vi "ControlCam-Final.vi"() -> ()   [LabVIEW 2014]
uses:
  <vilib>/vision/Vision Builder AI/API.llb/IVB Interface - VBAI Version.ctl
  <vilib>/vision/Vision Builder AI/API.llb/VBAI Interface - Get Inspection Image (By Name).vi
panel:
  out "Illegal?":bool
  out "Goal?":bool
  out "XY Graph":cluster{dbl[], dbl[]}[](graph)
  out "Ymovement":dbl
  out "X movefromcenter":dbl
  out "THETA case(deg)":dbl
  out "Defence 2 X":dbl format="%_4g"
  out "Defence 2 Y":dbl format="%_4g"
  in  "Kick":bool
  out "Defender 2":bool
  in  "Reset":bool
  out "Defender 1":bool
  out "Defenders":dbl
  out "MatchBall?":bool
  out "No.OfMatchball":dbl
  out "No.OfKicker":dbl
  out "Kicker There ?":bool
  out "Defence 1 Y":dbl format="%_4g"
  out "Defence 1 X":dbl format="%_4g"
  out "MatchBall Y":dbl format="%_4g"
  out "MatchBallX":dbl format="%_4g"
  out "Kicker Y":dbl format="%_4g"
  out "Kicker X":dbl format="%_4g"
  out "Image":T1(plugin-control)
  in  "stop":bool
  # "Manish's Free Kick Kicker"
  # "Co-ordinates in Centimeters"
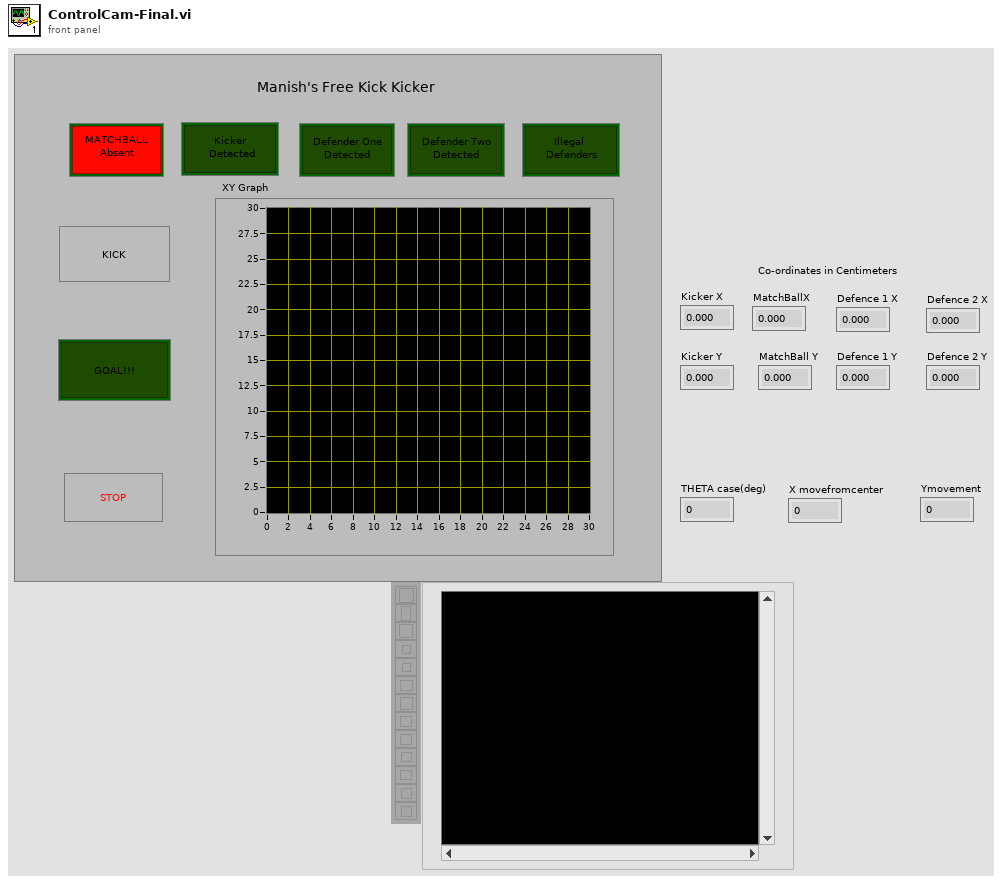
[diagram p1: front panel]
types:
  T1 = typedef "IMAQ Image.ctl" = refnum<image>
  T2 = typedef "Image Type" = u32
  T3 = typedef "IVB Interface - VBAI Version.ctl" = u16
  T4 = typedef "VBAIInterface.ctl" = refnum<k21>
  T5 = cluster{"PASS/FAIL Flag":bool, "Numeric Measurement":dbl, "String Measurement":string, "Report Text":string}[]
  T6 = cluster{"PASS/FAIL Flag":bool, "Numeric Measurement":dbl, "String Measurement":string, "Report Text":string}
  T7 = cluster{"m":dbl, "MatchBallX":dbl, "type":dbl, "MatchBallY":dbl}
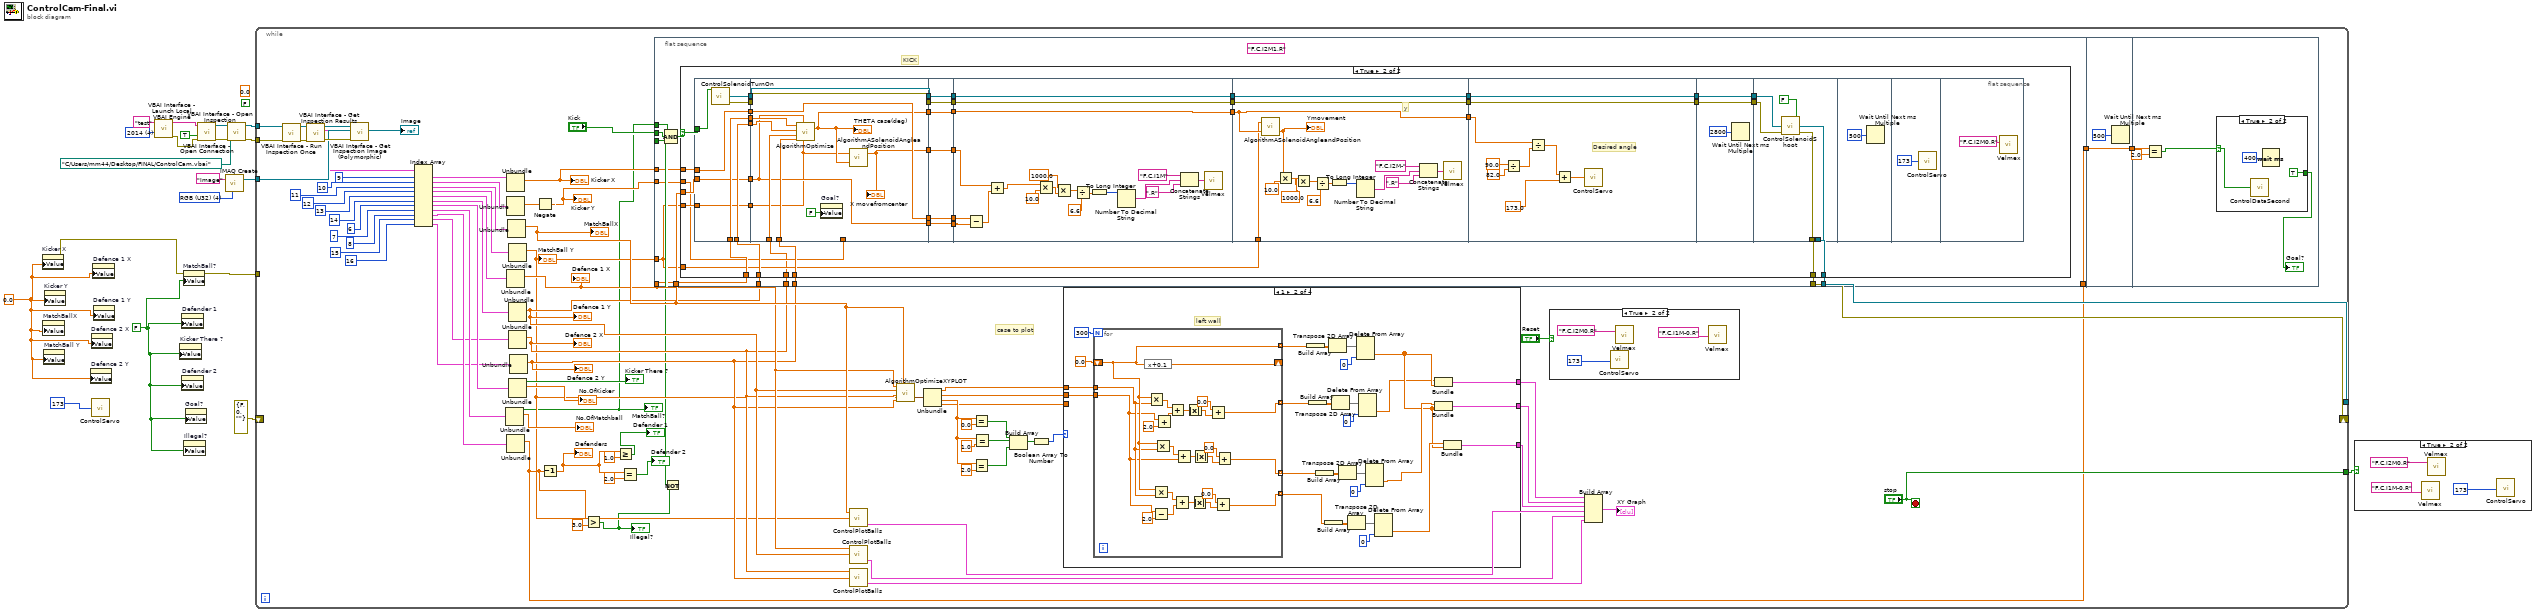
[diagram p0: block diagram]
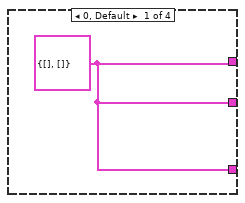
[diagram p3: hidden frame]
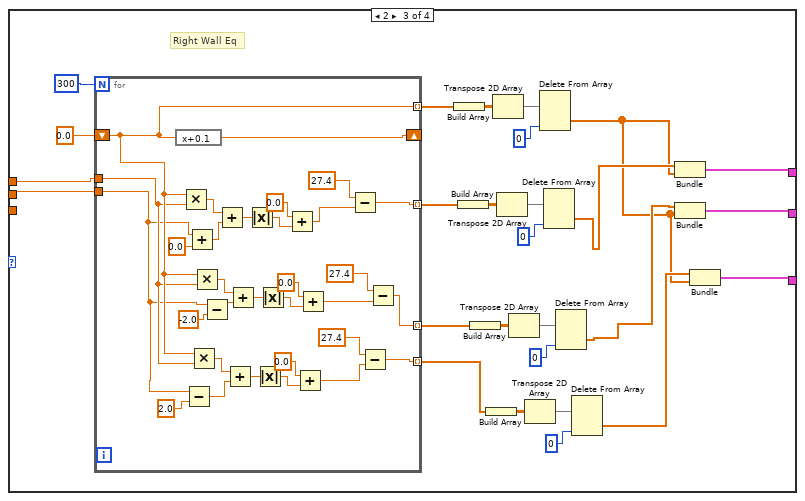
[diagram p4: hidden frame]
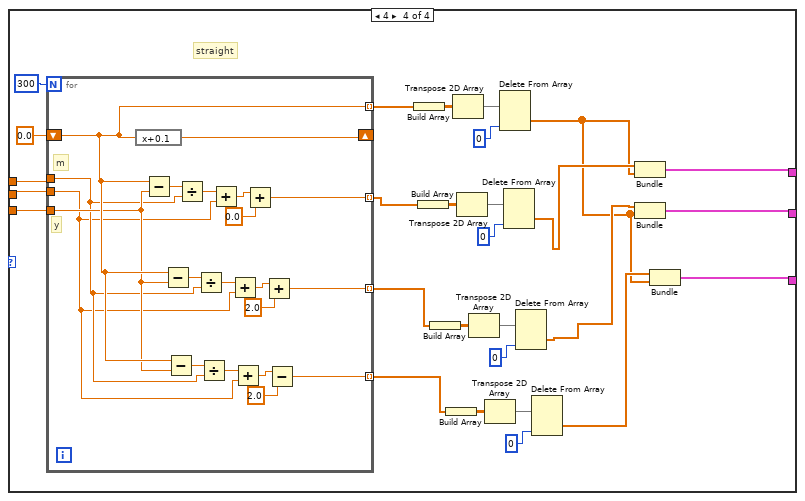
[diagram p5: hidden frame]
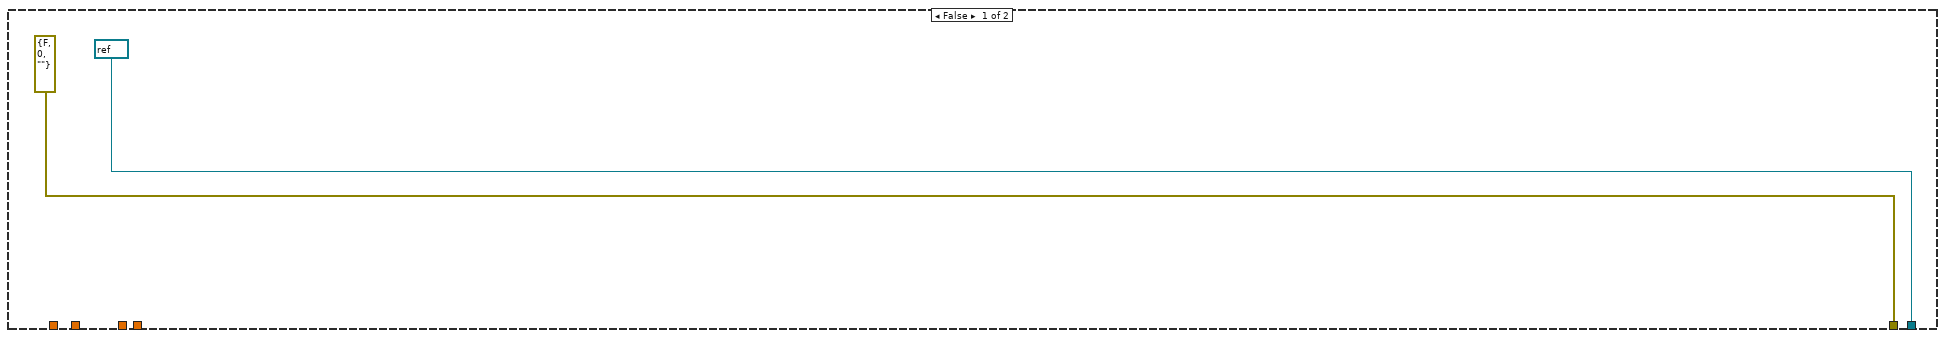
[diagram p6: hidden frame]
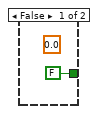
[diagram p7: hidden frame]
diagram:
  (unwired) FALSE
  (unwired) 0.0
  w3 = 0.0 ("Kicker X")
  w1 = FALSE
  w9 = T2 4 items=["Grayscale (U8)", "Grayscale (I16)", "Grayscale (SGL)", "Complex (CSG)", "RGB (U32)", "HSL (U32)", "RGB (U64)", "Grayscale (U16)"] ("Image Type")
  w17 = T3 4 items=["2010", "2011", "2012", "2013", "2014"] ("Engine Version")
  n1 = property on="Kicker X" class="DigNum (strict)"("Value"=w3) -> (error out=w4:errorcluster)  [unwired: 2 in, 1 out]
  n2 = property on="MatchBallX" class="DigNum (strict)"("Value"=w3) -> ()  [unwired: 2 in, 2 out]
  n3 = property on="MatchBall Y" class="DigNum (strict)"("Value"=w3) -> ()  [unwired: 2 in, 2 out]
  n4 = property on="Kicker Y" class="DigNum (strict)"("Value"=w3) -> ()  [unwired: 2 in, 2 out]
  n5 = property on="Defence 2 Y" class="DigNum (strict)"("Value"=w3) -> ()  [unwired: 2 in, 2 out]
  n6 = property on="Defence 2 X" class="DigNum (strict)"("Value"=w3) -> ()  [unwired: 2 in, 2 out]
  n7 = call "ControlServo.vi"("position"=u8 173) -> ()
  n8 = property on="Defence 1 X" class="DigNum (strict)"("Value"=w3) -> ()  [unwired: 2 in, 2 out]
  n9 = property on="Defence 1 Y" class="DigNum (strict)"("Value"=w3) -> ()  [unwired: 2 in, 2 out]
  n10 = call <vilib>:"VBAI Interface - Launch Local VBAI Engine.vi"("Engine Version"=w17, "Local VBAI Engine Name"="test") -> ("error out"=w8:errorcluster, "Session Name Out"=w18:string)  [unwired: 8 in]
  n11 = property on="Kicker There ?" class="Bool (strict)"("Value"=w1) -> ()  [unwired: 2 in, 2 out]
  n12 = property on="Defender 1" class="Bool (strict)"("Value"=w1) -> ()  [unwired: 2 in, 2 out]
  n13 = property on="Defender 2" class="Bool (strict)"("Value"=w1) -> ()  [unwired: 2 in, 2 out]
  n14 = property on="MatchBall?" class="Bool (strict)"(error in=w4, "Value"=w1) -> (error out=w7:errorcluster)  [unwired: 1 in, 1 out]
  n15 = property on="Illegal?" class="Bool (strict)"("Value"=w1) -> ()  [unwired: 2 in, 2 out]
  n16 = property on="Goal?" class="Bool (strict)"("Value"=w1) -> ()  [unwired: 2 in, 2 out]
  n17 = call <vilib>:"VBAI Interface - Open Connection.vi"("error in"=w8, "Force Connection (False)"=TRUE, "Session In"=w18) -> ("error out"=w16:errorcluster, "Session Out"=w15:T4)  [unwired: 7 in]
  n18 = call "IMAQ Create"("Image Name"="Image", "Image Type"=w9) -> ("New Image"=w11:T1)  [unwired: 3 in, 1 out]
  n19 = call <vilib>:"VBAI Interface - Open Inspection.vi"("error in"=w16, "Path"=path "C:/Users/mm44/Desktop/FINAL/ControlCam.vbai", "Session In"=w15) -> ("error out"=w12:errorcluster, "Session Out"=w13:T4)  [unwired: 7 in]
  n20 = while {
    tunnel: w13 -> [w98]
    tunnel: w12 -> [w97]
    tunnel: w11 -> [w94]
    tunnel: w7 -> [_]
    shift-right: [w57] -> _
    shift-left: errorcluster {"status"=FALSE, "code"=0, "source"=""} ("error out") -> [_]
    tunnel: [w58] -> _
    tunnel: ["stop"] -> w5
    stop <- "stop" stop-if-true
    # "case to plot"
    n21 = call <vilib>:"VBAI Interface - Run Inspection Once.vi"("error in"=w97, "Session In"=w98) -> ("error out"=w100:errorcluster, "Session Out"=w99:T4)  [unwired: 8 in]
    n22 = call <vilib>:"VBAI Interface - Get Inspection Results.vi"("error in"=w100, "Session In"=w99) -> ("error out"=w95:errorcluster, "Step Results"=w92:T5, "Session Out"=w96:T4)  [unwired: 3 in, 4 out]
    n23 = call-poly <vilib>:"VBAI Interface - Get Inspection Image (Polymorphic).vi"("error in"=w95, "Image Dest"=w94, "Session In"=w96) -> ("Image Dst Out"=→"Image":T1)  [unwired: 5 in, 3 out]
    n24 = Index Array(array=w92, index #1=9 ("index"), index #2=10 ("index"), index #3=11 ("index"), index #4=12 ("index"), index #5=13 ("index"), index #6=14 ("index"), index #7=6 ("index"), index #8=7 ("index"), index #9=8 ("index"), index #10=15 ("index"), index #11=16 ("index")) -> (element #1=w91:T6, element #2=w89:T6, element #3=w82:T6, element #4=w81:T6, element #5=w80:T6, element #6=w79:T6, element #7=w77:T6, element #8=w73:T6, element #9=w71:T6, element #10=w62:T6, element #11=w61:T6)
    n25 = Unbundle(w73) -> ("PASS/FAIL Flag"=w25:bool, "Numeric Measurement"=→"No.OfMatchball":dbl)  [unwired: 2 out]
    "MatchBall?" <- w25
    n26 = Unbundle(w91) -> ("Numeric Measurement"=w52:dbl)  [unwired: 3 out]
    "Kicker X" <- w52
    n27 = Unbundle(w89) -> ("Numeric Measurement"=w88:dbl)  [unwired: 3 out]
    n28 = Unbundle(w80) -> ("Numeric Measurement"=w36:dbl)  [unwired: 3 out]
    "Defence 1 X" <- w36
    n29 = Unbundle(w71) -> ("Numeric Measurement"=w23:dbl)  [unwired: 3 out]
    n30 = Unbundle(w82) -> ("Numeric Measurement"=w37:dbl)  [unwired: 3 out]
    "MatchBallX" <- w37
    n31 = Unbundle(w81) -> ("Numeric Measurement"=w32:dbl)  [unwired: 3 out]
    "MatchBall Y" <- w32
    n32 = Unbundle(w79) -> ("Numeric Measurement"=w35:dbl)  [unwired: 3 out]
    "Defence 1 Y" <- w35
    n33 = Unbundle(w62) -> ("Numeric Measurement"=w34:dbl)  [unwired: 3 out]
    "Defence 2 X" <- w34
    n34 = Unbundle(w77) -> ("PASS/FAIL Flag"=→"Kicker There ?":bool, "Numeric Measurement"=→"No.OfKicker":dbl)  [unwired: 2 out]
    n35 = Unbundle(w61) -> ("Numeric Measurement"=w33:dbl)  [unwired: 3 out]
    "Defence 2 Y" <- w33
    n36 = Negate(x=w88) -> (-x=w51:dbl)
    "Kicker Y" <- w51
    n37 = Decrement(x=w23) -> (x-1=w65:dbl)
    "Defenders" <- w65
    n38 = Greater?(x=w23, y=3.0) -> (0:w22:bool)
    "Illegal?" <- w22
    n39 = Greater Or Equal?(x=w65, y=1.0) -> (x >= y?=→"Defender 1":bool)
    n40 = Equal?(x=w65, y=2.0) -> (x = y?=→"Defender 2":bool)
    n41 = flat-sequence {
      tunnel: "Kick" -> [w260]
      tunnel: [w272] -> w58
      tunnel: [w271] -> w57
      tunnel: w52 -> [w270]
      tunnel: w51 -> [w269]
      tunnel: w37 -> [w268]
      tunnel: w32 -> [w267]
      tunnel: w36 -> [w266]
      tunnel: w35 -> [w265]
      tunnel: w34 -> [w264]
      tunnel: w33 -> [w263]
      tunnel: w23 -> [w262]
      tunnel: [w262] -> w26
      tunnel: w25 -> [w261]
      tunnel: w21 -> [w258]
      tunnel: [w397] -> w27
      tunnel: w26 -> [w397]
      tunnel: w27 -> [w402]
      frame #0 {
        (unwired) "F,C,I2M1,R" ("string")
        # "KICK"
        n42 = Compound Arithmetic op=AND(w261, w260, w258) -> (w259:bool)
        n43 = case shown="True" w259 {
          selector: w259 -> [_ w311]
          tunnel: w268 -> [_ w315]
          tunnel: w267 -> [_ w281]
          tunnel: w270 -> [_ w314]
          tunnel: [refnum<k21> refnum ("task out") w313] -> w272
          tunnel: [errorcluster {"status"=FALSE, "code"=0, "source"=""} ("error out") w312] -> w271
          tunnel: w266 -> [_ w301]
          tunnel: w265 -> [_ w300]
          tunnel: w264 -> [_ w275]
          tunnel: w263 -> [_ w298]
          tunnel: w269 -> [_ w277]
          tunnel: w267 -> [_ w276]
          frame False {
          }
          frame True {
            n44 = flat-sequence {
              tunnel: w314 -> [w317]
              tunnel: w315 -> [w318]
              tunnel: [w318] -> w306
              tunnel: [w317] -> w305
              tunnel: w311 -> [w323]
              tunnel: [w322] -> w304
              tunnel: [w321] -> w303
              tunnel: [w320] -> w302
              tunnel: w301 -> [w320]
              tunnel: w300 -> [w319]
              tunnel: [w319] -> w299
              tunnel: [w316] -> w282
              tunnel: w281 -> [w316]
              tunnel: w306 -> [w328]
              tunnel: [w328] -> w297
              tunnel: w305 -> [w333]
              tunnel: [w333] -> w296
              tunnel: w304 -> [w335]
              tunnel: [w335] -> w294
              tunnel: w303 -> [w334]
              tunnel: [w334] -> w292
              tunnel: w302 -> [w332]
              tunnel: w299 -> [w331]
              tunnel: w275 -> [w330]
              tunnel: w298 -> [w329]
              tunnel: [w327] -> w290
              tunnel: w282 -> [w324]
              tunnel: [w326] -> w280
              tunnel: w277 -> [_]
              tunnel: w297 -> [w337]
              tunnel: w296 -> [w341]
              tunnel: [w341] -> w295
              tunnel: w294 -> [w340]
              tunnel: [w340] -> w293
              tunnel: w292 -> [w339]
              tunnel: [w339] -> w291
              tunnel: w290 -> [w338]
              tunnel: [w338] -> w289
              tunnel: [w337] -> w283
              tunnel: w280 -> [w336]
              tunnel: [w336] -> w279
              tunnel: w295 -> [w347]
              tunnel: [w350] -> w288
              tunnel: w293 -> [w350]
              tunnel: [w349] -> w286
              tunnel: w291 -> [w349]
              tunnel: [w348] -> w284
              tunnel: w289 -> [w348]
              tunnel: w283 -> [w346]
              tunnel: w279 -> [w343]
              tunnel: w288 -> [w376]
              tunnel: [w376] -> w287
              tunnel: w286 -> [w375]
              tunnel: [w375] -> w285
              tunnel: w284 -> [w362]
              tunnel: [w362] -> w278
              tunnel: w276 -> [w361]
              tunnel: [w385] -> w309
              tunnel: w287 -> [w385]
              tunnel: [w384] -> w307
              tunnel: w285 -> [w384]
              tunnel: w278 -> [w381]
              tunnel: [w388] -> w310
              tunnel: w309 -> [w388]
              tunnel: [w387] -> w308
              tunnel: w307 -> [w387]
              tunnel: [w392] -> w313
              tunnel: [w391] -> w312
              tunnel: w310 -> [w390]
              tunnel: w308 -> [w389]
              frame #0 {
                n45 = call "ControlSolenoidTurnOn.vi"("On?"=w323) -> ("error out"=w321:errorcluster, "task out"=w322:refnum<k21>)
              }
              frame #1 {
                n46 = call "AlgorithmOptimize.vi"("MatchBallY"=w324, "MatchBallX"=w328, "D2 Y COM"=w329, "D2 X COM"=w330, "D1Y COM"=w331, "D1 X COM 2"=w332) -> ("THETA"=w327:dbl)  [unwired: 1 in]
                "THETA case(deg)" <- w327
                n47 = property on="Goal?" class="Bool (strict)"("Value"=FALSE ("Goal?")) -> ()  [unwired: 2 in, 2 out]
                n48 = call "AlgorithmASolenoidAngleandPosition.vi"("Theta in degrees"=w327, "MartchBall Y"=w324) -> ("X movefromcenter"=w326:dbl)  [unwired: 1 out]
                "X movefromcenter" <- w326
              }
              frame #2 {
              }
              frame #3 {
                n49 = Subtract(x=w347, y=w346) -> (x-y=w344:dbl)
                n50 = Add(x=w343, y=w344) -> (x+y=w345:dbl)
                n51 = Multiply(x=w345, y=10.0) -> (x*y=w357:dbl)
                n52 = Multiply(x=1000.0, y=w357) -> (x*y=w355:dbl)
                n53 = Divide(x=w355, y=6.6) -> (x/y=w342:dbl)
                n54 = To Long Integer(number=w342) -> (32bit integer=w353:i32)
                n55 = Number To Decimal String(number=w353) -> (decimal integer string=w352:string)  [unwired: 1 in]
                n56 = Concatenate Strings("F,C,I1M" ("string"), w352, ",R" ("string")) -> (w351:string)
                n57 = call "Velmex.Vi"("Command String"=w351) -> ()  [unwired: 6 in]
              }
              frame #4 {
                # "y"
                n58 = call "AlgorithmASolenoidAngleandPosition.vi"("Theta in degrees"=w362, "MartchBall Y"=w361) -> ("Ymovement"=w363:dbl)  [unwired: 1 out]
                "Ymovement" <- w363
                n59 = Multiply(x=w363, y=10.0) -> (x*y=w367:dbl)
                n60 = Multiply(x=1000.0, y=w367) -> (x*y=w369:dbl)
                n61 = Divide(x=w369, y=6.6) -> (x/y=w371:dbl)
                n62 = To Long Integer(number=w371) -> (32bit integer=w372:i32)
                n63 = Number To Decimal String(number=w372) -> (decimal integer string=w373:string)  [unwired: 1 in]
                n64 = Concatenate Strings("F,C,I2M-" ("string"), w373, ",R" ("string")) -> (w374:string)
                n65 = call "Velmex.Vi"("Command String"=w374) -> ()  [unwired: 6 in]
              }
              frame #5 {
                # "Desired angle"
                n66 = Divide(x=90.0, y=82.0) -> (x/y=w380:dbl)
                n67 = Divide(x=w381, y=w380) -> (x/y=w379:dbl)
                n68 = Add(x=w379, y=173.0) -> (x+y=w377:dbl)
                n69 = call "ControlServo.vi"("position"=w377) -> ()
              }
              frame #6 {
                n70 = Wait Until Next ms Multiple(millisecond multiple=u32 2800) -> ()  [unwired: 1 out]
              }
              frame #7 {
                n71 = call "ControlSolenoidShoot.vi"("error in"=w389, "task/channels in"=w390, "On?"=FALSE) -> ("error out"=w391:errorcluster, "task out"=w392:refnum<k21>)  [unwired: 1 in]
              }
              frame #8 {
                n72 = Wait Until Next ms Multiple(millisecond multiple=u32 500) -> ()  [unwired: 1 out]
              }
              frame #9 {
                n73 = call "ControlServo.vi"("position"=173) -> ()
              }
              frame #10 {
                n74 = call "Velmex.Vi"("Command String"="F,C,I2M0,R" ("Y 2")) -> ()  [unwired: 6 in]
              }
            }
          }
        }
      }
      frame #1 {
        n75 = Wait Until Next ms Multiple(millisecond multiple=u32 500) -> ()  [unwired: 1 out]
      }
      frame #2 {
        n76 = Equal?(x=w402, y=2.0) -> (x = y?=w400:bool)
        n77 = case shown="True" w400 {
          selector: w400 -> [_ w404]
          tunnel: [FALSE TRUE] -> w399
          frame False {
            (unwired) 0.0
          }
          frame True {
            n78 = call "ControlDataSecond.vi"("Boolean"=w404) -> ()  [unwired: 2 in]
            n79 = Wait (ms)(milliseconds to wait=u32 400) -> ()  [unwired: 1 out]
          }
        }
        "Goal?" <- w399
      }
    }
    n80 = Not(x=w22) -> (.not. x?=w21:bool)
    n81 = call "ControlPlotBalls.vi"("Y-center"=w32, "x-center"=w37) -> ("XY Graph"=w55:cluster{dbl[], dbl[]})
    n82 = call "ControlPlotBalls.vi"("Y-center"=w35, "x-center"=w36) -> ("XY Graph"=w54:cluster{dbl[], dbl[]})
    n83 = call "ControlPlotBalls.vi"("Y-center"=w33, "x-center"=w34) -> ("XY Graph"=w50:cluster{dbl[], dbl[]})
    n84 = call "AlgorithmOptimizeXYPLOT.vi"("MatchBallY"=w32, "MatchBallX"=w37, "D2 Y COM"=w33, "D2 X COM"=w34, "D1Y COM"=w35, "D1 X COM 2"=w36) -> ("Plot"=w49:T7)  [unwired: 1 out]
    n85 = Unbundle(w49) -> ("m"=w40:dbl, "MatchBallX"=w39:dbl, "type"=w45:dbl, "MatchBallY"=w38:dbl)
    n86 = Equal?(x=w45, y=0.0) -> (x = y?=w46:bool)
    n87 = Equal?(x=w45, y=2.0) -> (x = y?=w42:bool)
    n88 = Equal?(x=w45, y=1.0) -> (x = y?=w43:bool)
    n89 = Build Array(w46, w43, w42) -> (w47:bool[])
    n90 = Boolean Array To Number(Boolean array=w47) -> (number=w41:u32)
    n91 = case shown="1" w41 {
      tunnel: w40 -> [_ w107 w156 w217]
      tunnel: w39 -> [_ w106 w155 w216]
      tunnel: w38 -> [_ _ _ w218]
      tunnel: [w101 w105 w154 w212] -> w29
      tunnel: [w101 w104 w153 w211] -> w30
      tunnel: [w101 w103 w152 w210] -> w31
      frame 0, Default {
        w101 = cluster{dbl[], dbl[]} {[], []}
      }
      frame 1 {
        # "left wall"
        n92 = for {
          N: 300 -> [_]
          shift-right: [w151] -> _
          shift-left: 0.0 -> [w138]
          tunnel: [w138] -> w126 mode=indexing
          tunnel: [w146] -> w119 mode=indexing
          tunnel: [w142] -> w114 mode=indexing
          tunnel: [w136] -> w110 mode=indexing
          tunnel: w107 -> [w137]
          tunnel: w106 -> [w131]
          n93 = expression code="x+0.1"(w138) -> (w151:dbl)
          n94 = Multiply(x=w138, y=w137) -> (x*y=w150:dbl)
          n95 = Multiply(x=w138, y=w137) -> (x*y=w132:dbl)
          n96 = Subtract(x=w131, y=2.0 ("x")) -> (x-y=w130:dbl)
          n97 = Multiply(x=w138, y=w137) -> (x*y=w135:dbl)
          n98 = Add(x=w131, y=2.0 ("x")) -> (x+y=w134:dbl)
          n99 = Add(x=w150, y=w134) -> (x+y=w149:dbl)
          n100 = Add(x=w132, y=w130) -> (x+y=w139:dbl)
          n101 = Add(x=w135, y=w131) -> (x+y=w145:dbl)
          n102 = Absolute Value(x=w149) -> (abs(x)=w148:dbl)
          n103 = Absolute Value(x=w139) -> (abs(x)=w140:dbl)
          n104 = Absolute Value(x=w145) -> (abs(x)=w144:dbl)
          n105 = Add(x=0.0, y=w148) -> (x+y=w146:dbl)
          n106 = Add(x=0.0, y=w140) -> (x+y=w136:dbl)
          n107 = Add(x=0.0, y=w144) -> (x+y=w142:dbl)
        }
        n108 = Build Array(w126) -> (w125:dbl[][])
        n109 = Build Array(w119) -> (w120:dbl[][])
        n110 = Build Array(w114) -> (w116:dbl[][])
        n111 = Build Array(w110) -> (w113:dbl[][])
        n112 = Transpose 2D Array(2D array=w125) -> (transposed array=w124:dbl[][])
        n113 = Transpose 2D Array(2D array=w120) -> (transposed array=w121:dbl[][])
        n114 = Transpose 2D Array(2D array=w116) -> (transposed array=w117:dbl[][])
        n115 = Transpose 2D Array(2D array=w113) -> (transposed array=w112:dbl[][])
        n116 = Delete From Array(array=w124, index (col)=0 ("disabled index (col)")) -> (deleted portion=w108:dbl[])  [unwired: 2 in, 1 out]
        n117 = Delete From Array(array=w121, index (col)=0 ("disabled index (col)")) -> (deleted portion=w102:dbl[])  [unwired: 2 in, 1 out]
        n118 = Delete From Array(array=w117, index (col)=0 ("disabled index (col)")) -> (deleted portion=w115:dbl[])  [unwired: 2 in, 1 out]
        n119 = Delete From Array(array=w112, index (col)=0 ("disabled index (col)")) -> (deleted portion=w109:dbl[])  [unwired: 2 in, 1 out]
        n120 = Bundle(w102, w108) -> (w105:cluster{dbl[], dbl[]})  [unwired: 1 in]
        n121 = Bundle(w115, w108) -> (w104:cluster{dbl[], dbl[]})  [unwired: 1 in]
        n122 = Bundle(w109, w108) -> (w103:cluster{dbl[], dbl[]})  [unwired: 1 in]
      }
      frame 2 {
        # "Right Wall Eq"
        n123 = for {
          N: 300 -> [_]
          shift-right: [w209] -> _
          shift-left: 0.0 -> [w198]
          tunnel: [w198] -> w176 mode=indexing
          tunnel: [w196] -> w169 mode=indexing
          tunnel: [w188] -> w163 mode=indexing
          tunnel: [w189] -> w159 mode=indexing
          tunnel: w156 -> [w197]
          tunnel: w155 -> [w181]
          n124 = expression code="x+0.1"(w198) -> (w209:dbl)
          n125 = Multiply(x=w198, y=w197) -> (x*y=w187:dbl)
          n126 = Subtract(x=w181, y=2.0 ("x")) -> (x-y=w184:dbl)
          n127 = Add(x=w181, y=0.0 ("x")) -> (x+y=w186:dbl)
          n128 = Multiply(x=w198, y=w197) -> (x*y=w182:dbl)
          n129 = Multiply(x=w198, y=w197) -> (x*y=w205:dbl)
          n130 = Subtract(x=w181, y=-2.0 ("x")) -> (x-y=w180:dbl)
          n131 = Add(x=w187, y=w186) -> (x+y=w208:dbl)
          n132 = Add(x=w182, y=w184) -> (x+y=w199:dbl)
          n133 = Add(x=w205, y=w180) -> (x+y=w204:dbl)
          n134 = Absolute Value(x=w208) -> (abs(x)=w207:dbl)
          n135 = Absolute Value(x=w199) -> (abs(x)=w200:dbl)
          n136 = Absolute Value(x=w204) -> (abs(x)=w203:dbl)
          n137 = Add(x=0.0, y=w207) -> (x+y=w194:dbl)
          n138 = Add(x=0.0, y=w200) -> (x+y=w190:dbl)
          n139 = Add(x=0.0, y=w203) -> (x+y=w191:dbl)
          n140 = Subtract(x=27.4, y=w194) -> (x-y=w196:dbl)
          n141 = Subtract(x=27.4, y=w190) -> (x-y=w189:dbl)
          n142 = Subtract(x=27.4, y=w191) -> (x-y=w188:dbl)
        }
        n143 = Build Array(w176) -> (w175:dbl[][])
        n144 = Build Array(w169) -> (w170:dbl[][])
        n145 = Build Array(w163) -> (w166:dbl[][])
        n146 = Build Array(w159) -> (w162:dbl[][])
        n147 = Transpose 2D Array(2D array=w175) -> (transposed array=w174:dbl[][])
        n148 = Transpose 2D Array(2D array=w170) -> (transposed array=w171:dbl[][])
        n149 = Transpose 2D Array(2D array=w166) -> (transposed array=w167:dbl[][])
        n150 = Transpose 2D Array(2D array=w162) -> (transposed array=w161:dbl[][])
        n151 = Delete From Array(array=w174, index (col)=0 ("disabled index (col)")) -> (deleted portion=w157:dbl[])  [unwired: 2 in, 1 out]
        n152 = Delete From Array(array=w171, index (col)=0 ("disabled index (col)")) -> (deleted portion=w164:dbl[])  [unwired: 2 in, 1 out]
        n153 = Delete From Array(array=w167, index (col)=0 ("disabled index (col)")) -> (deleted portion=w165:dbl[])  [unwired: 2 in, 1 out]
        n154 = Delete From Array(array=w161, index (col)=0 ("disabled index (col)")) -> (deleted portion=w158:dbl[])  [unwired: 2 in, 1 out]
        n155 = Bundle(w164, w157) -> (w154:cluster{dbl[], dbl[]})  [unwired: 1 in]
        n156 = Bundle(w165, w157) -> (w153:cluster{dbl[], dbl[]})  [unwired: 1 in]
        n157 = Bundle(w158, w157) -> (w152:cluster{dbl[], dbl[]})  [unwired: 1 in]
      }
      frame 4 {
        # "straight"
        n158 = for {
          N: 300 -> [_]
          shift-right: [w257] -> _
          shift-left: 0.0 -> [w243]
          tunnel: [w243] -> w235 mode=indexing
          tunnel: w217 -> [w241]
          tunnel: w216 -> [w240]
          tunnel: w218 -> [w242]
          tunnel: [w252] -> w215 mode=indexing
          tunnel: [w239] -> w214 mode=indexing
          tunnel: [w238] -> w213 mode=indexing
          # "y"
          # "m"
          n159 = expression code="x+0.1"(w243) -> (w257:dbl)
          n160 = Subtract(x=w243, y=w242) -> (x-y=w256:dbl)
          n161 = Subtract(x=w243, y=w242) -> (x-y=w248:dbl)
          n162 = Subtract(x=w243, y=w242) -> (x-y=w247:dbl)
          n163 = Divide(x=w256, y=w241) -> (x/y=w255:dbl)
          n164 = Divide(x=w248, y=w241) -> (x/y=w249:dbl)
          n165 = Divide(x=w247, y=w241) -> (x/y=w246:dbl)
          n166 = Add(x=w255, y=w240) -> (x+y=w254:dbl)
          n167 = Add(x=w249, y=w240) -> (x+y=w250:dbl)
          n168 = Add(x=w246, y=w240) -> (x+y=w245:dbl)
          n169 = Add(x=w254, y=0.0) -> (x+y=w252:dbl)
          n170 = Add(x=w250, y=2.0) -> (x+y=w239:dbl)
          n171 = Subtract(x=w245, y=2.0) -> (x-y=w238:dbl)
        }
        n172 = Build Array(w235) -> (w234:dbl[][])
        n173 = Build Array(w215) -> (w229:dbl[][])
        n174 = Build Array(w214) -> (w226:dbl[][])
        n175 = Build Array(w213) -> (w223:dbl[][])
        n176 = Transpose 2D Array(2D array=w234) -> (transposed array=w233:dbl[][])
        n177 = Transpose 2D Array(2D array=w229) -> (transposed array=w230:dbl[][])
        n178 = Transpose 2D Array(2D array=w226) -> (transposed array=w227:dbl[][])
        n179 = Transpose 2D Array(2D array=w223) -> (transposed array=w222:dbl[][])
        n180 = Delete From Array(array=w233, index (col)=0 ("disabled index (col)")) -> (deleted portion=w219:dbl[])  [unwired: 2 in, 1 out]
        n181 = Delete From Array(array=w230, index (col)=0 ("disabled index (col)")) -> (deleted portion=w224:dbl[])  [unwired: 2 in, 1 out]
        n182 = Delete From Array(array=w227, index (col)=0 ("disabled index (col)")) -> (deleted portion=w225:dbl[])  [unwired: 2 in, 1 out]
        n183 = Delete From Array(array=w222, index (col)=0 ("disabled index (col)")) -> (deleted portion=w220:dbl[])  [unwired: 2 in, 1 out]
        n184 = Bundle(w224, w219) -> (w212:cluster{dbl[], dbl[]})  [unwired: 1 in]
        n185 = Bundle(w225, w219) -> (w211:cluster{dbl[], dbl[]})  [unwired: 1 in]
        n186 = Bundle(w220, w219) -> (w210:cluster{dbl[], dbl[]})  [unwired: 1 in]
      }
    }
    n187 = case shown="True" "Reset" {
      frame False {
      }
      frame True {
        n188 = call "ControlServo.vi"("position"=173) -> ()
        n189 = call "Velmex.Vi"("Command String"="F,C,I2M0,R" ("Y 2")) -> ()  [unwired: 6 in]
        n190 = call "Velmex.Vi"("Command String"="F,C,I1M-0,R" ("X 2")) -> ()  [unwired: 6 in]
      }
    }
    n191 = Build Array(w29, w30, w31, w55, w54, w50) -> (→"XY Graph":cluster{dbl[], dbl[]}[])
  }
  n192 = case shown="True" w5 {
    frame False {
    }
    frame True {
      n193 = call "Velmex.Vi"("Command String"="F,C,I1M-0,R" ("X 2")) -> ()  [unwired: 6 in]
      n194 = call "Velmex.Vi"("Command String"="F,C,I2M0,R" ("Y 2")) -> ()  [unwired: 6 in]
      n195 = call "ControlServo.vi"("position"=173) -> ()
    }
  }
